vi "Configure Directory.vi"(8 "error in (no error)":errorcluster, 9 "Folder Operation (0: Select Folder)":i32(ring) items=["Select Folder", "Make New Folder", "Remove Folder"], 10 "Folder ()":string, 11 "VISA resource name":refnum<visa-resource-name>) -> (0 "error out":errorcluster, 3 "VISA resource name out":refnum<visa-resource-name>)   [LabVIEW 2013, in "Agilent 3446X Series.lvlib"]
doc: "Configures folder settings."
uses:
  Agilent 3446X Series.lvlib
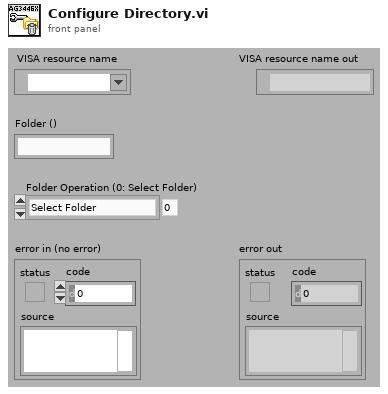
[diagram p1: front panel]
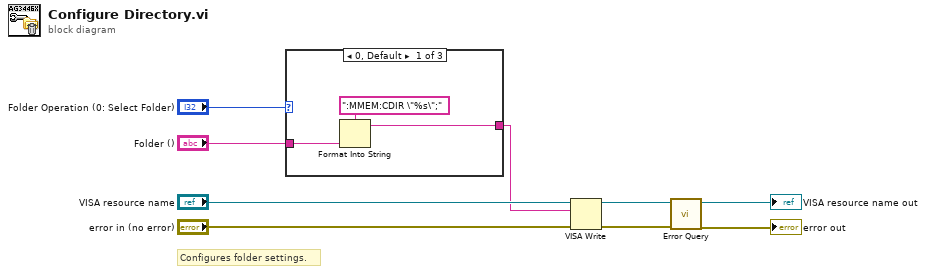
[diagram p0: block diagram]
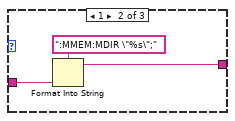
[diagram p2: hidden frame]
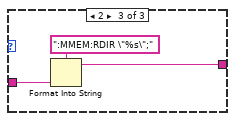
[diagram p3: hidden frame]
diagram:
  # "Configures folder settings."
  n1 = case shown="0, Default" "Folder Operation (0: Select Folder)" {
    tunnel: "Folder ()" -> [w11 w14 w17]
    tunnel: [w10 w13 w16] -> w1
    frame 0, Default {
      n2 = Format Into String(format string=":MMEM:CDIR \"%s\";", w11) -> (resulting string=w10:string)  [unwired: 2 in, 1 out]
    }
    frame 1 {
      n3 = Format Into String(format string=":MMEM:MDIR \"%s\";", w14) -> (resulting string=w13:string)  [unwired: 2 in, 1 out]
    }
    frame 2 {
      n4 = Format Into String(format string=":MMEM:RDIR \"%s\";", w17) -> (resulting string=w16:string)  [unwired: 2 in, 1 out]
    }
  }
  n5 = VISA Write(VISA resource name="VISA resource name", write buffer=w1, error in (no error)="error in (no error)") -> (VISA resource name out=w7:refnum<visa-resource-name>, error out=w6:errorcluster)  [unwired: 1 out]
  n6 = call "Error Query.vi"("error in (no error)"=w6, "VISA resource name"=w7) -> ("error out"=→"error out":errorcluster, "VISA resource name out"=→"VISA resource name out":refnum<visa-resource-name>)  [unwired: 8 out]
